vi "motor and torque test.vi"() -> ()   [LabVIEW 2025]
uses:
  Classes/Stepper/Path Mode.ctl
  Classes/Stepper/Stepper.lvclass
  Classes/USB IO/USB IO.lvclass
  Classes/Torque Transducer/Torque Transducer.lvclass
  Classes/USB IO/Relay Line.ctl
  <vilib>/Handler Framework/CmdQueue/Enqueue Single.vi
  <vilib>/Handler Framework/Handler Framework.lvlib
panel:
  out "error out 3":errorcluster
  out "data value":dbl
  out "error out 2":errorcluster
  in  "Clear error":bool
  out "error out":errorcluster
  out "Angle":dbl
  in  "Tab Control":T1(tab)
  in  "Parameters":u32[](array[numeric]) format="%.0x"
  out "Hex Result":u32[](array[numeric]) format="%.0x"
  out "Decimal Result":u32[](array[numeric])
  in  "Check Params":bool
  out "Bin Result":u32[](array[numeric]) format="%.0b"
  in  "Radix":u16(ring)=5 items=["Decimal"=0, "Binary"=3, "Hex"=5]
  in  "Write Params":bool
  in  "Parameters to Write":u32[](array[numeric]) format="%.0x"
  in  "Values to Write":u32[](array[numeric])
  in  "Clear Motor Error":bool
  in  "Quick Stop":bool
  in  "CCW?":bool
  in  "JOG":bool
  in  "Path Number":i32
  in  "Run Path":bool
  in  "Write Path":bool
  in  "Path Cluster":T3={"Path Number"=0, "Path Mode"=enum."Position Mode", "Relative?"=enum."Relative", "Angle"=180.0, "Velocity [rpm]"=10, "Acceleration [ms/krpm]"=10, "Deceleration [ms/krpm]"=10, "Pause Time [ms]"=50}
  out "Waveform Chart 2":dbl(graph)
  out "Waveform Chart":dbl(graph)
  in  "Brake":bool
  # "ERRORS:"
  # "CHECK PARAMETERS:"
  # "WRITE PARAMETERS:"
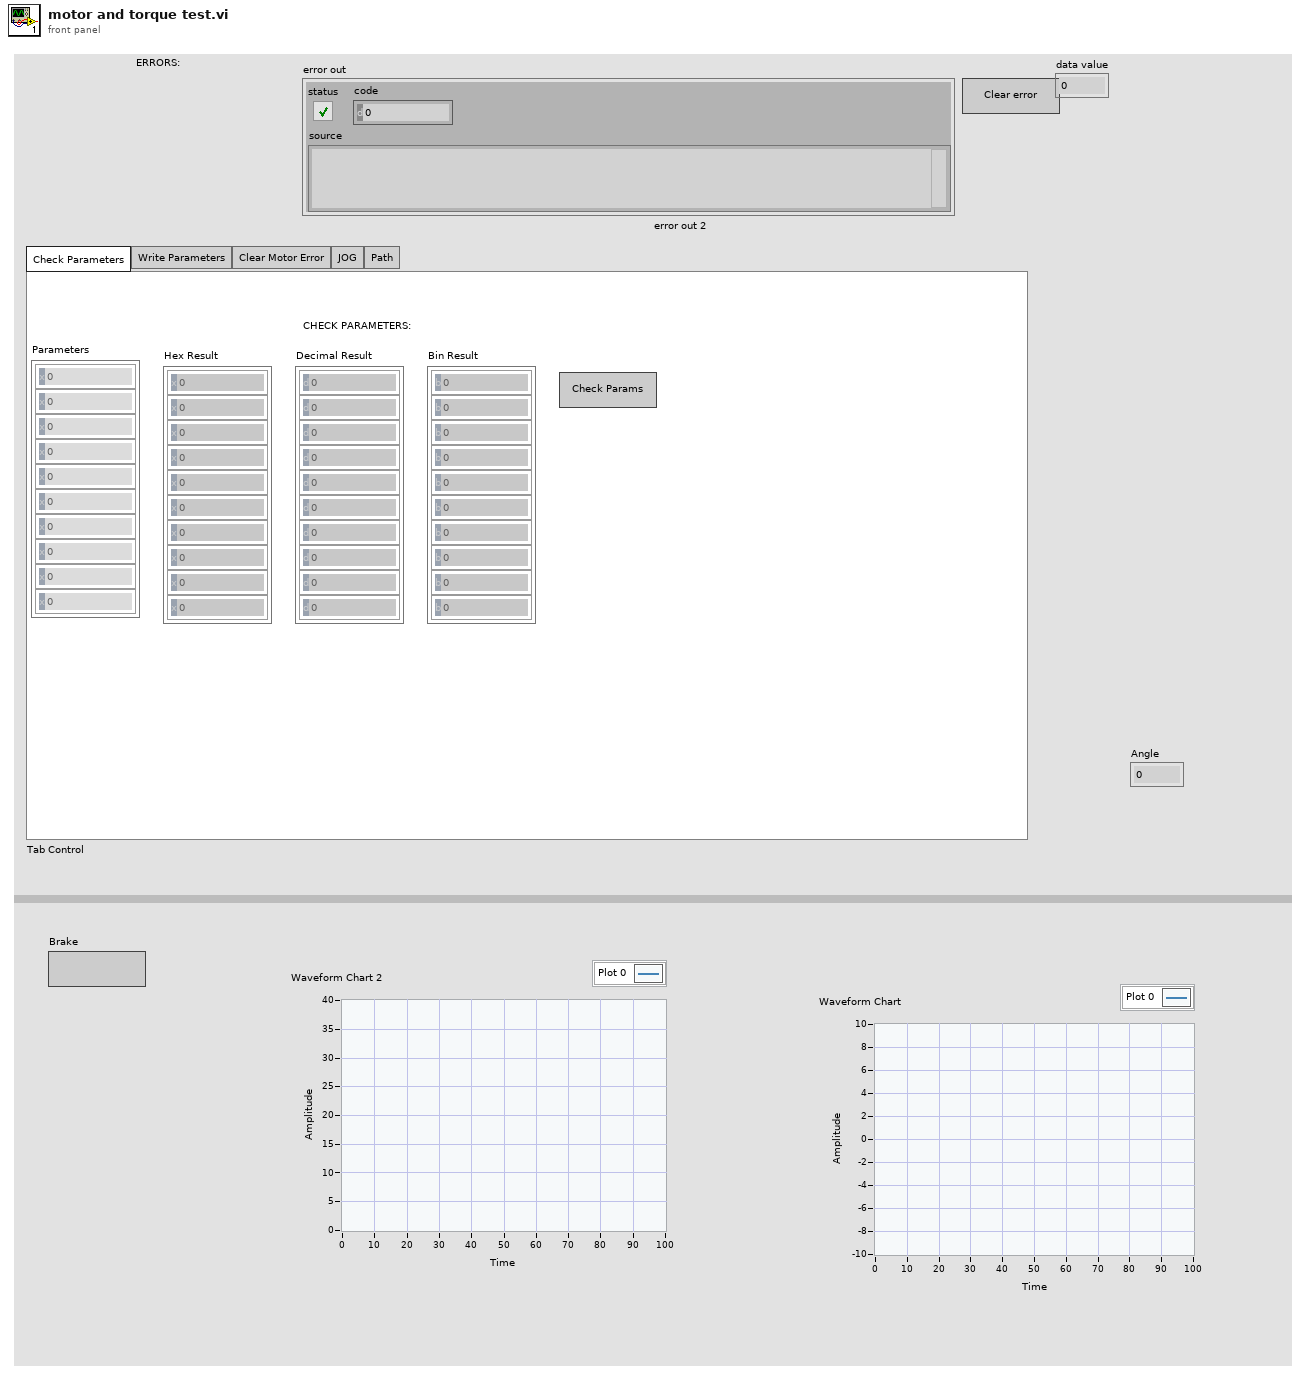
[diagram p1: front panel]
types:
  T1 = enum32{"Check Parameters", "Write Parameters", "Clear Motor Error", "JOG", "Path"}
  T2 = typedef "Path Mode.ctl" = enum16{"Position Mode", "Velocity Mode", "Homing Mode"}
  T3 = cluster{"Path Number":i32, "Path Mode":T2, "Relative?":enum16{"Relative", "Absolute"}, "Angle":dbl, "Velocity [rpm]":i32, "Acceleration [ms/krpm]":i32, "Deceleration [ms/krpm]":i32, "Pause Time [ms]":i32}
  T4 = typedef "Relay Line.ctl" = enum16{"Brake Relay", "PS Relay"}
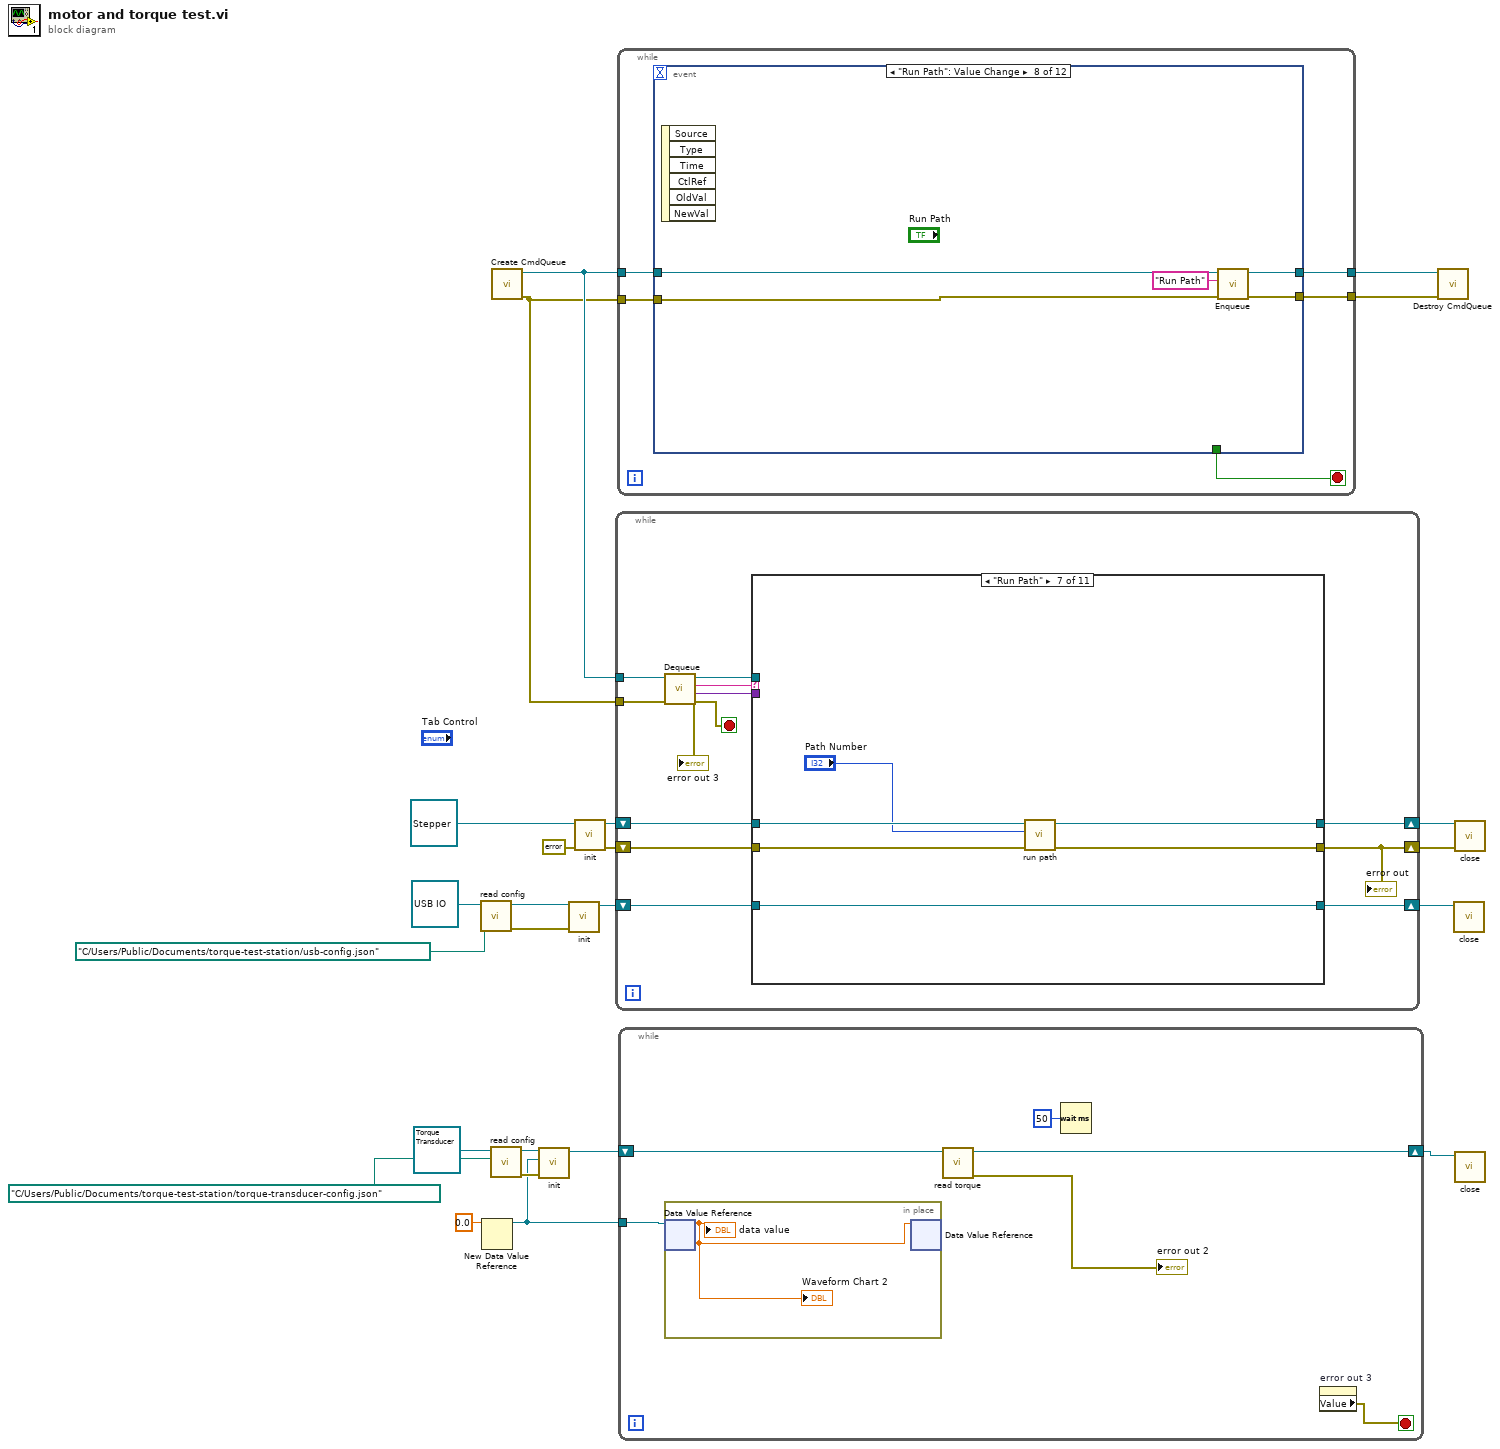
[diagram p0: block diagram]
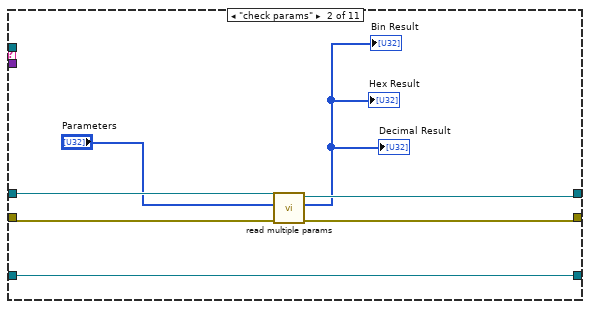
[diagram p3: hidden frame]
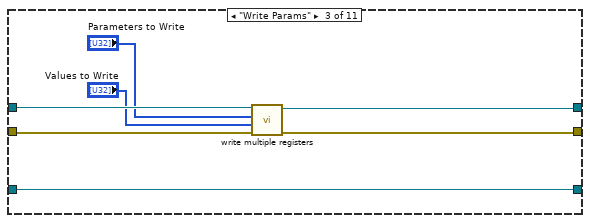
[diagram p4: hidden frame]
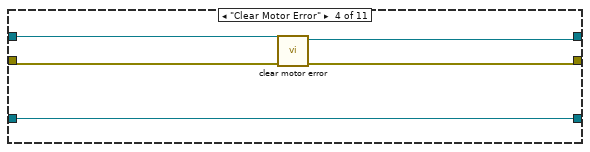
[diagram p5: hidden frame]
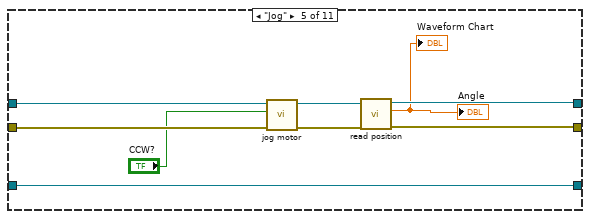
[diagram p6: hidden frame]
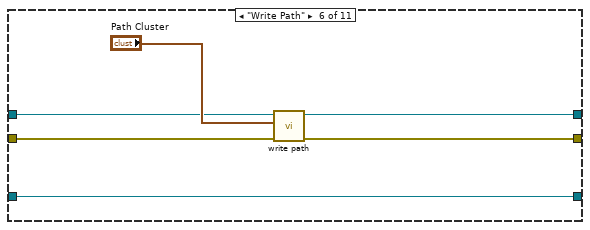
[diagram p7: hidden frame]
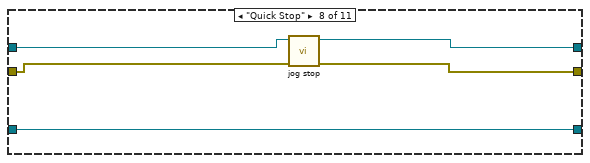
[diagram p8: hidden frame]
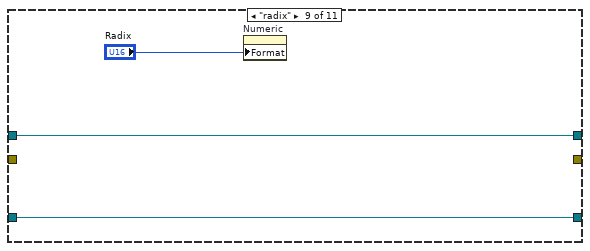
[diagram p9: hidden frame]
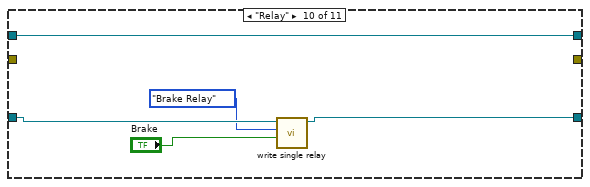
[diagram p10: hidden frame]
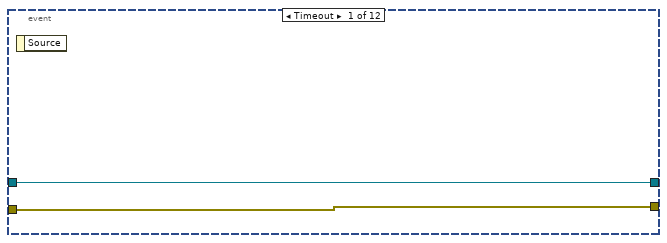
[diagram p12: hidden frame]
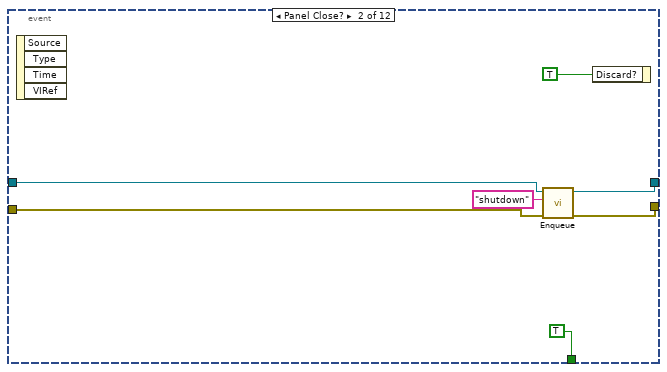
[diagram p13: hidden frame]
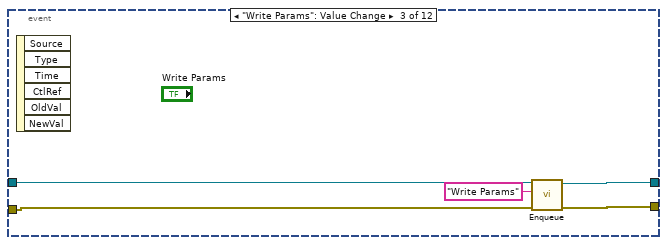
[diagram p14: hidden frame]
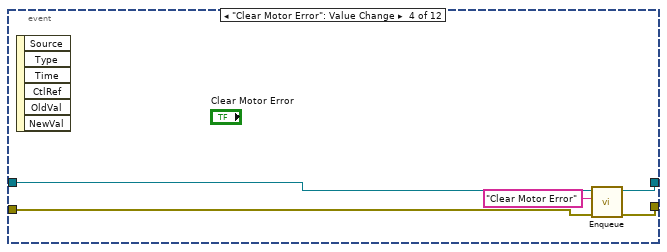
[diagram p15: hidden frame]
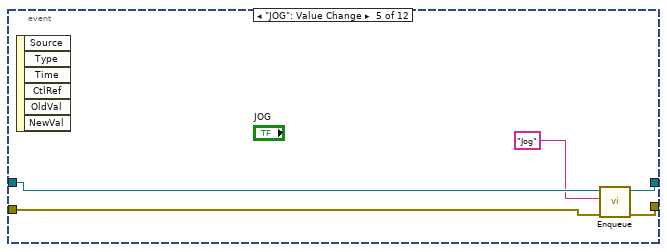
[diagram p16: hidden frame]
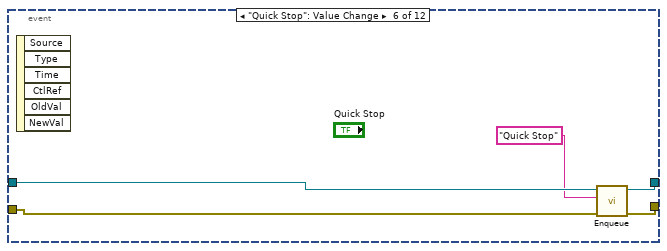
[diagram p17: hidden frame]
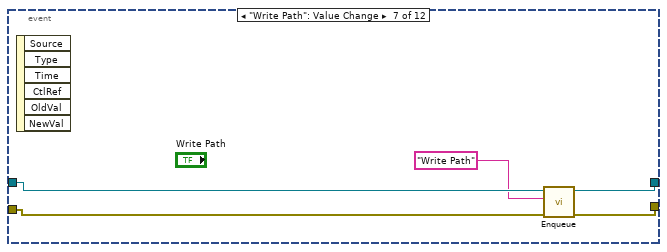
[diagram p18: hidden frame]
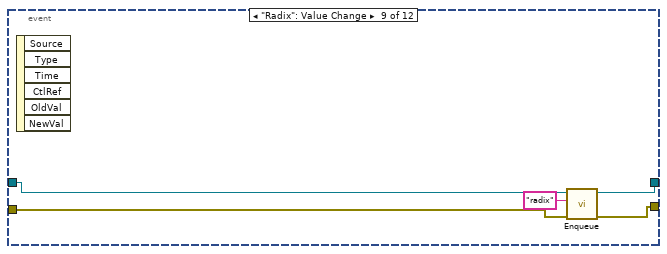
[diagram p19: hidden frame]
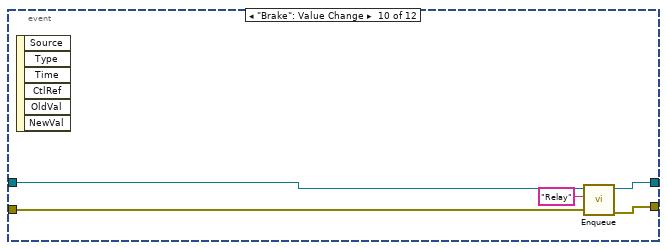
[diagram p20: hidden frame]
diagram:
  n1 = call-dynamic "read config.vi"("config file path"=path "C:/Users/Public/Documents/torque-test-station/usb-config.json", "USB IO in"=refnum<class "USB IO.lvclass"> refnum ("USB IO.lvclass")) -> ("error out"=w11:errorcluster, "USB IO out"=w12:refnum<class "USB IO.lvclass">)  [unwired: 8 in]
  n2 = New Data Value Reference(data value=0.0) -> (data value reference=w2:refnum<data-value>)  [unwired: 1 in, 1 out]
  n3 = call-dynamic "read config.vi"("Path"=path "C:/Users/Public/Documents/torque-test-station/torque-transducer-config.json", "Torque Transducer in"=refnum<class "Torque Transducer.lvclass"> refnum ("Torque Transducer.lvclass")) -> ("error out"=w5:errorcluster, "Torque Transducer out"=w6:refnum<class "Torque Transducer.lvclass">)  [unwired: 8 in]
  n4 = call <vilib>:"Create CmdQueue.vi"() -> ("error out"=w21:errorcluster, "CmdQueue out"=w24:refnum<queue>)  [unwired: 10 in]
  n5 = call-dynamic "init.vi"("error in (no error)"=w5, "Torque Value"=w2, "Torque Transducer in"=w6) -> ("Torque Transducer out"=w3:refnum<class "Torque Transducer.lvclass">)  [unwired: 7 in, 1 out]
  n6 = call-dynamic "init.vi"("error in (no error)"=w11, "USB IO in"=w12) -> ("USB IO out"=w10:refnum<class "USB IO.lvclass">)  [unwired: 8 in, 1 out]
  n7 = call-dynamic "init.vi"("error in (no error)"=errorcluster {"status"=FALSE, "code"=0, "source"=""}, "Stepper in"=refnum<class "Stepper.lvclass"> refnum ("Stepper.lvclass")) -> ("error out"=w19:errorcluster, "Stepper out"=w20:refnum<class "Stepper.lvclass">)  [unwired: 8 in]
  n8 = while {
    tunnel: w24 -> [w36]
    tunnel: w21 -> [w35]
    shift-right: [w28] -> w18
    shift-left: w19 -> [w29]
    shift-right: [w27] -> w17
    shift-left: w20 -> [w30]
    shift-right: [w25] -> w9
    shift-left: w10 -> [w26]
    stop <- w32 stop-if-true
    n9 = call <vilib>:"Dequeue.vi"("error in (no error)"=w35, "CmdQueue in"=w36) -> ("error out"=w32:errorcluster, "value"=w33:variant, "cmd"=w34:string, "CmdQueue out"=w31:refnum<queue>)  [unwired: 5 in, 1 out]
    "error out 3" <- w32
    n10 = case shown="\"Run Path\"" w34 {
      tunnel: w33 -> [_ _ _ _ _ _ _ _ _ _ _]
      tunnel: w31 -> [_ _ _ _ _ _ _ _ _ _ _]
      tunnel: w30 -> [w38 w46 w52 w58 w67 w69 w78 w84 w86 w88 w94]
      tunnel: w29 -> [w39 w42 w51 w57 w66 w70 w76 w83 _ _ _]
      tunnel: [w39 w43 w47 w55 w60 w71 w74 w81 _ _ _] -> w28
      tunnel: [w38 w44 w48 w56 w61 w72 w75 w82 w86 w88 w94] -> w27
      tunnel: w26 -> [w37 w40 w53 w54 w64 w68 w79 w80 w85 w92 w93]
      tunnel: [w37 w40 w53 w54 w64 w68 w79 w80 w85 w89 w93] -> w25
      frame "", Default {
      }
      frame "check params" {
        n11 = call-dynamic "read multiple params.vi"("error in (no error)"=w42, "Parameters"="Parameters", "Stepper in"=w46) -> ("error out"=w43:errorcluster, "Hex Result"=→"Hex Result" →"Decimal Result" →"Bin Result":u32[], "Stepper out"=w44:refnum<class "Stepper.lvclass">)  [unwired: 6 in]
      }
      frame "Write Params" {
        n12 = call-dynamic "write multiple registers.vi"("error in (no error)"=w51, "register values"="Values to Write", "addresses"="Parameters to Write", "Stepper in"=w52) -> ("error out"=w47:errorcluster, "Stepper out"=w48:refnum<class "Stepper.lvclass">)  [unwired: 6 in]
      }
      frame "Clear Motor Error" {
        n13 = call-dynamic "clear motor error.vi"("error in (no error)"=w57, "Stepper in"=w58) -> ("error out"=w55:errorcluster, "Stepper out"=w56:refnum<class "Stepper.lvclass">)  [unwired: 8 in]
      }
      frame "Jog" {
        n14 = call-dynamic "jog motor.vi"("error in (no error)"=w66, "CCW? (T)"="CCW?", "Stepper in"=w67) -> ("error out"=w62:errorcluster, "Stepper out"=w63:refnum<class "Stepper.lvclass">)  [unwired: 7 in]
        n15 = call-dynamic "read position.vi"("error in (no error)"=w62, "Stepper in"=w63) -> ("error out"=w60:errorcluster, "Angle"=→"Angle" →"Waveform Chart":dbl, "Stepper out"=w61:refnum<class "Stepper.lvclass">)  [unwired: 7 in]
      }
      frame "Write Path" {
        n16 = call-dynamic "write path.vi"("error in (no error)"=w70, "Path Cluster"="Path Cluster", "Stepper in"=w69) -> ("error out"=w71:errorcluster, "Stepper out"=w72:refnum<class "Stepper.lvclass">)  [unwired: 7 in]
      }
      frame "Run Path" {
        n17 = call-dynamic "run path.vi"("error in (no error)"=w76, "Path Number"="Path Number", "Stepper in"=w78) -> ("error out"=w74:errorcluster, "Stepper out"=w75:refnum<class "Stepper.lvclass">)  [unwired: 7 in]
      }
      frame "Quick Stop" {
        n18 = call-dynamic "jog stop.vi"("error in (no error)"=w83, "Stepper in"=w84) -> ("error out"=w81:errorcluster, "Stepper out"=w82:refnum<class "Stepper.lvclass">)  [unwired: 8 in]
      }
      frame "radix" {
        n19 = property on="Numeric" class="DigNum (strict)"("Format"="Radix") -> ()  [unwired: 2 in, 2 out]
      }
      frame "Relay" {
        n20 = call-dynamic "write single relay.vi"("High/Low"="Brake", "Line Enum"=Relay_Line."Brake Relay", "USB IO in"=w92) -> ("USB IO out"=w89:refnum<class "USB IO.lvclass">)  [unwired: 7 in, 1 out]
      }
      frame "clear error" {
      }
    }
    "error out" <- w28
  }
  n21 = while {
    tunnel: w24 -> [w99]
    tunnel: [w98] -> w23
    tunnel: [w97] -> w22
    tunnel: w21 -> [w96]
    stop <- w95 stop-if-true
    n22 = event shown="[7] \"Run Path\": Value Change" {
      selector: _ -> [_ _ _ _ _ _ _ _ _ _ _ _]
      dyn-events: _ -> [_ _ _ _ _ _ _ _ _ _ _ _]
      timeout: _ -> [_ _ _ _ _ _ _ _ _ _ _ _]
      tunnel: w99 -> [w101 w104 w110 w116 w120 w126 w130 w135 w141 w146 w151 w156]
      tunnel: [w101 w106 w113 w118 w123 w127 w133 w138 w143 w148 w153 w158] -> w98
      tunnel: [w100 w105 w112 w117 w122 w128 w132 w137 w142 w147 w152 w157] -> w97
      tunnel: w96 -> [w100 w103 w111 w115 w121 w125 w131 w136 w140 w145 w150 w155]
      tunnel: [_ TRUE _ _ _ _ _ _ _ _ _ _] -> w95
      event Timeout {
        n23 = event-data() -> ()  [unwired: 1 in, 1 out]
      }
      event Panel Close? {
        n24 = event-data() -> ()  [unwired: 1 in, 4 out]
        n25 = call-poly <vilib>:"Enqueue.vi"("error in (no error)"=w103, "Command"="shutdown", "CmdQueue in"=w104) -> ("error out"=w105:errorcluster, "CmdQueue out"=w106:refnum<queue>)  [unwired: 7 in]
        n26 = event-data("Discard?"=TRUE) -> ()  [unwired: 1 in, 1 out]
      }
      event "Write Params": Value Change {
        n27 = event-data() -> ()  [unwired: 1 in, 6 out]
        n28 = call-poly <vilib>:"Enqueue.vi"("error in (no error)"=w111, "Command"="Write Params", "CmdQueue in"=w110) -> ("error out"=w112:errorcluster, "CmdQueue out"=w113:refnum<queue>)  [unwired: 7 in]
      }
      event "Clear Motor Error": Value Change {
        n29 = event-data() -> ()  [unwired: 1 in, 6 out]
        n30 = call-poly <vilib>:"Enqueue.vi"("error in (no error)"=w115, "Command"="Clear Motor Error", "CmdQueue in"=w116) -> ("error out"=w117:errorcluster, "CmdQueue out"=w118:refnum<queue>)  [unwired: 7 in]
      }
      event "JOG": Value Change {
        n31 = event-data() -> ()  [unwired: 1 in, 6 out]
        n32 = call-poly <vilib>:"Enqueue.vi"("error in (no error)"=w121, "Command"="Jog", "CmdQueue in"=w120) -> ("error out"=w122:errorcluster, "CmdQueue out"=w123:refnum<queue>)  [unwired: 7 in]
      }
      event "Quick Stop": Value Change {
        n33 = event-data() -> ()  [unwired: 1 in, 6 out]
        n34 = call-poly <vilib>:"Enqueue.vi"("error in (no error)"=w125, "Command"="Quick Stop", "CmdQueue in"=w126) -> ("error out"=w128:errorcluster, "CmdQueue out"=w127:refnum<queue>)  [unwired: 7 in]
      }
      event "Write Path": Value Change {
        n35 = event-data() -> ()  [unwired: 1 in, 6 out]
        n36 = call-poly <vilib>:"Enqueue.vi"("error in (no error)"=w131, "Command"="Write Path", "CmdQueue in"=w130) -> ("error out"=w132:errorcluster, "CmdQueue out"=w133:refnum<queue>)  [unwired: 7 in]
      }
      event "Run Path": Value Change {
        n37 = event-data() -> ()  [unwired: 1 in, 6 out]
        n38 = call-poly <vilib>:"Enqueue.vi"("error in (no error)"=w136, "Command"="Run Path", "CmdQueue in"=w135) -> ("error out"=w137:errorcluster, "CmdQueue out"=w138:refnum<queue>)  [unwired: 7 in]
      }
      event "Radix": Value Change {
        n39 = event-data() -> ()  [unwired: 1 in, 6 out]
        n40 = call-poly <vilib>:"Enqueue.vi"("error in (no error)"=w140, "Command"="radix", "CmdQueue in"=w141) -> ("error out"=w142:errorcluster, "CmdQueue out"=w143:refnum<queue>)  [unwired: 7 in]
      }
      event "Brake": Value Change {
        n41 = event-data() -> ()  [unwired: 1 in, 6 out]
        n42 = call-poly <vilib>:"Enqueue.vi"("error in (no error)"=w145, "Command"="Relay", "CmdQueue in"=w146) -> ("error out"=w147:errorcluster, "CmdQueue out"=w148:refnum<queue>)  [unwired: 7 in]
      }
      event "Check Params", "Parameters": Value Change {
        n43 = event-data() -> ()  [unwired: 1 in, 6 out]
        n44 = call-poly <vilib>:"Enqueue.vi"("error in (no error)"=w150, "Command"="check params", "CmdQueue in"=w151) -> ("error out"=w152:errorcluster, "CmdQueue out"=w153:refnum<queue>)  [unwired: 7 in]
      }
      event "Clear error": Value Change {
        n45 = event-data() -> ()  [unwired: 1 in, 6 out]
        n46 = call-poly <vilib>:"Enqueue.vi"("error in (no error)"=w155, "Command"="clear error", "CmdQueue in"=w156) -> ("error out"=w157:errorcluster, "CmdQueue out"=w158:refnum<queue>)  [unwired: 7 in]
      }
    }
  }
  n47 = while {
    shift-right: [w163] -> w1
    shift-left: w3 -> [w164]
    tunnel: w2 -> [w161]
    stop <- w160 stop-if-true
    n48 = in-place {
      n49 = in-place-dvr #1(w161) -> (w165:dbl)  [unwired: 1 out]
      "data value" <- w165
      "Waveform Chart 2" <- w165
      n50 = in-place-dvr #1(w165) -> ()  [unwired: 2 out]
    }
    n51 = call-dynamic "read torque.vi"("Torque Transducer in"=w164) -> ("error out"=→"error out 2":errorcluster, "Torque Transducer out"=w163:refnum<class "Torque Transducer.lvclass">)  [unwired: 9 in]
    n52 = Wait (ms)(milliseconds to wait=u32 50) -> ()  [unwired: 1 out]
    n53 = property on="error out 3" class="Clust (strict)"() -> ("Value"=w160:errorcluster)  [unwired: 2 in, 2 out]
  }
  n54 = call <vilib>:"Destroy CmdQueue.vi"("error in (no error)"=w22, "CmdQueue in"=w23) -> ()  [unwired: 9 in, 1 out]
  n55 = call-dynamic "close.vi"("USB IO in"=w9) -> ()  [unwired: 9 in, 2 out]
  n56 = call-dynamic "close.vi"("error in (no error)"=w18, "Stepper in"=w17) -> ()  [unwired: 8 in, 2 out]
  n57 = call-dynamic "close.vi"("Torque Transducer in"=w1) -> ()  [unwired: 9 in, 2 out]
